vi "Aquire Z-Stack.vi"(4 "Acquisition Progres Bar":refnum<vi>, 6 "Move Relative Increment":string, 7 "queue in":refnum<queue>, 8 "error in (no error)":errorcluster, 9 "Number of slices":i32, 10 "PI ID in":i32, 11 "pDataBuffer":u16[](array[numeric])) -> (0 "error out":errorcluster, 3 "PI ID out":i32, 5 "queue out":refnum<queue>)   [LabVIEW 2020]
uses:
  _Controls/Logging Queue Cluster.ctl
  _Controls/Tweezertron Ctrl Refs.ctl
  _Controls/Confocal Controls.ctl
  _Controls/iFlex.ctl
  _Controls/PIFOC Position.ctl
  _Controls/Manlight Controls.ctl
  _Controls/Exp Params.ctl
  _Controls/Image Thresholds.ctl
  _Controls/Spots.ctl
  <vilib>/Platform/TimedLoop/XDataNode/timing_clust.ctl
  <vilib>/Platform/TimedLoop/XDataNode/nitl_modes.ctl
  <vilib>/Platform/TimedLoop/XDataNode/wakeup.ctl
  _Globals/Global Controls.vi
  <vilib>/Platform/TimedLoop/XDataNode/XDataNode.xnode
  <vilib>/Platform/TimedLoop/XDataNode/XDNodeRunTimeDep.lvlib
panel:
  # "Made this vi time critical on Nov 21st 2018"
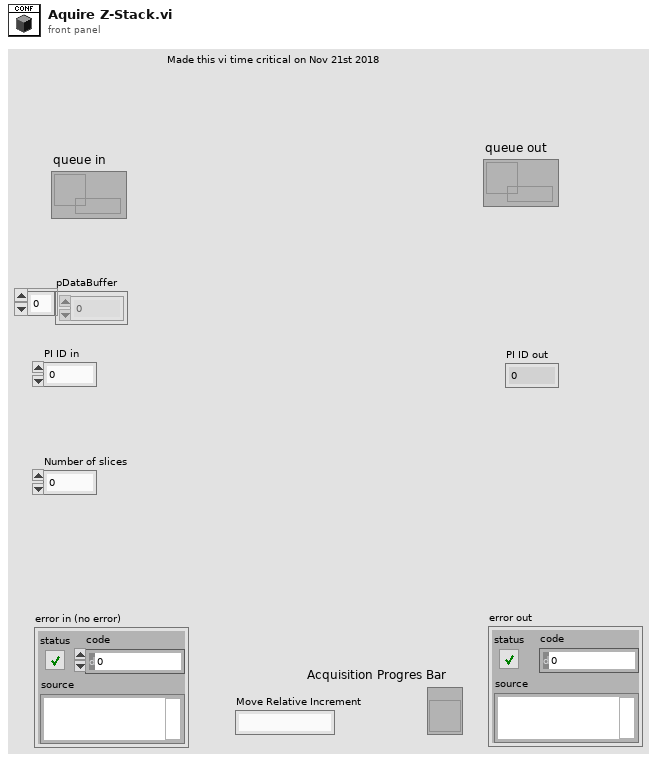
[diagram p1: front panel]
types:
  T1 = typedef "XDNodeRunTimeDep.lvlib/timing_clust.ctl" = cluster{"Expected End [f-1]":u64, "Actual End [f-1]":u64, "Finished Late? [f-1]":bool, "Expected End [i-1]":u64, "Actual End [i-1]":u64, "Finished Late? [i-1]":bool, "Expected Start [i]":u64, "Actual Start [i]":u64, "Expected Start [f]":u64, "Actual Start [f]":u64, "Source Name":string, "Structure Name":string, "Period":i64, "Deadline":i64, "Offset":i64, "Start":i64, "Priority":i32, "Timeout":i32, "Mode":T2, "Wakeup Reason":T3, "Error":errorcluster, "Source Type":string, "Secondary Source Type":string, "Global End Time":u64, "Global Start Time":u64, "Frame Duration":u64, "Iteration Duration":u64, "Assigned CPU":i32, "I/O Scan Engine Mode":u32}
  T2 = typedef "XDNodeRunTimeDep.lvlib/nitl_modes.ctl" = enum32{"No Change", "Process missed periods, maintain original phase", "Discard missed periods, maintain original phase", "Process missed periods, ignore original phase", "Discard missed periods, ignore original phase"}
  T3 = typedef "XDNodeRunTimeDep.lvlib/wakeup.ctl" = enum32{"Normal", "Aborted", "Asynchronous wakeup", "Timing source error", "Timed loop error", "Timeout"}
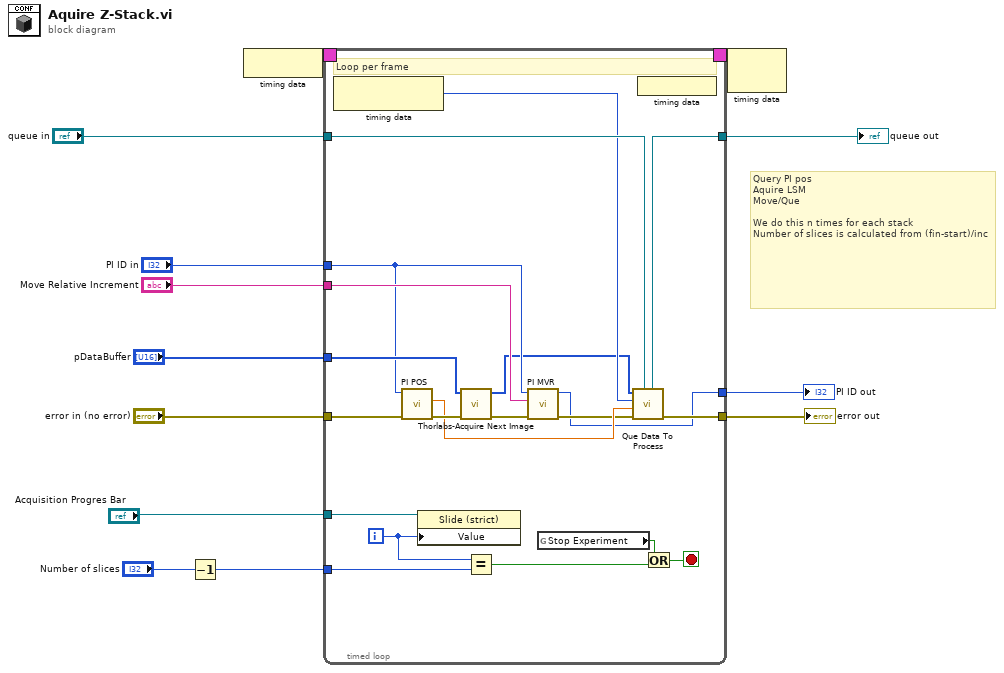
[diagram p0: block diagram]
diagram:
  # "Query PI pos\nAquire LSM\nMove/Que\n\nWe do this n times for each stack\nNumber of slices is calculated from (fin-start)/inc"
  n1 = Decrement(x="Number of slices") -> (x-1=w5:i32)
  n2 = node-c288() -> (w8:T1)
  n3 = timed-loop {
    tunnel: "pDataBuffer" -> [w33]
    tunnel: "error in (no error)" -> [w23]
    tunnel: [w29] -> w13
    tunnel: "PI ID in" -> [w21]
    tunnel: "Move Relative Increment" -> [w24]
    tunnel: "queue in" -> [w31]
    tunnel: "Acquisition Progres Bar" -> [w32]
    tunnel: [w30] -> w1
    timing: w8 -> [_]
    timing-out: [_] -> w7
    tunnel: w5 -> [w27]
    tunnel: [w17] -> w4
    i -> [w28]
    stop <- w14 stop-if-true
    # "Loop per frame"
    n4 = node-c288() -> (w26:i64)  [unwired: 1 in]
    n5 = call "PI POS.vi"("error in (no error)"=w23, "ID in"=w21) -> ("error out"=w22:errorcluster, "Position"=w19:dbl)  [unwired: 7 in, 1 out]
    n6 = property class="Slide (strict)"(reference=w32, "Value"=w28) -> ()  [unwired: 1 in, 2 out]
    n7 = call "Thorlabs-Acquire Next Image.vi"("error in (no error)"=w22, "pDataBuffer in"=w33) -> ("error out"=w25:errorcluster, "pDataBuffer out"=w20:u16[])  [unwired: 7 in, 1 out]
    n8 = Equal?(x=w28, y=w27) -> (x = y?=w15:bool)
    n9 = call "PI MVR.vi"("error in (no error)"=w25, "String"=w24, "PI ID in"=w21) -> ("error out"=w18:errorcluster, "PI ID out"=w17:i32)  [unwired: 6 in, 1 out]
    n10 = global read "Global Controls.vi" "Stop Experiment"() -> (w16:bool)
    n11 = call "Que Data To Process.vi"("queue in"=w31, "error in (no error)"=w18, "PIFOC Pos"=w19, "timestamp (nm)"=w26, "pDataBuffer in"=w20) -> ("error out"=w29:errorcluster, "queue out"=w30:refnum<queue>)  [unwired: 5 in]
    n12 = node-c288() -> ()  [unwired: 1 out]
    n13 = Or(x=w16, y=w15) -> (x .or. y?=w14:bool)
  }
  "error out" <- w13
  "PI ID out" <- w4
  "queue out" <- w1
  n14 = node-c288(w7) -> ()  [unwired: 1 out]
